vi "Get Assertion Status From Test Case.vi"(11 "Test Case Test Double in":refnum<class "Test Case Test Double.lvclass">) -> (2 "Message":string, 3 "Status":T1)   [LabVIEW 2020, in "LUnit Tests.lvlib" / "Compare Assertion Test.lvclass"]
uses:
  Compare Assertion Test.lvclass
  source/Framework/Result Classes/Assertion Result/Public/TypeDefs/Status.ctl
  Test Dummys/Test Case Test Double/Test Case Test Double.lvclass
  C:/Users/anton/Documents/GitHub/LUnit/source/Framework/Test Case/LUnit Test Case.lvclass
  source/Framework/Test Case/LUnit Test Case.lvclass/LUnit Test Case.ctl
  source/Framework/Result Classes/Test Case Result/Test Case Result.lvclass/Test Case Result.ctl
  source/Framework/Result Classes/Method Result/Method Result.lvclass/Method Result.ctl
  source/Framework/Result Classes/Assertion Result/Assertion Result.lvclass/Assertion Result.ctl
  source/Framework/Test Case/LUnit Test Case.lvclass
  source/Framework/Result Classes/Test Case Result/Test Case Result.lvclass
  source/Framework/Result Classes/Method Result/Method Result.lvclass
  source/Framework/Result Classes/Assertion Result/Assertion Result.lvclass
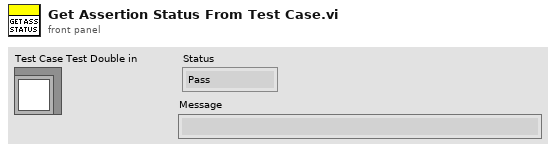
[diagram p1: front panel]
types:
  T1 = typedef "Assertion Result.lvclass/Status.ctl" = enum16{"Pass", "Fail", "Error", "Skipped", "Setup Error", "Broken", "Teardown Error"}
  T2 = map{string, refnum<class "Method Result.lvclass">}
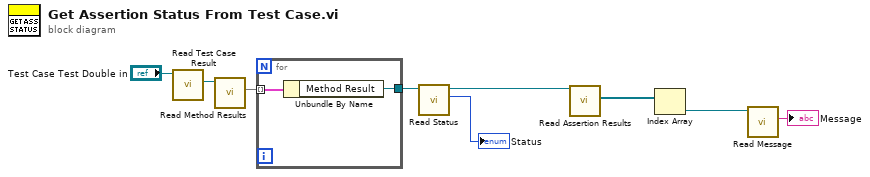
[diagram p0: block diagram]
diagram:
  n1 = call "Read Test Case Result.vi"("LUnit Test Case In"="Test Case Test Double in") -> ("Test Case Result"=w6:refnum<class "Test Case Result.lvclass">)  [unwired: 9 in, 1 out]
  n2 = call "Read Method Results.vi"("Test Case Result In"=w6) -> ("Method Results"=w7:T2)  [unwired: 9 in, 1 out]
  n3 = for {
    tunnel: [w11] -> w8
    tunnel: w7 -> [w10] mode=indexing
    n4 = Unbundle By Name(w10) -> ("Method Result"=w11:refnum<class "Method Result.lvclass">)
  }
  n5 = call "Read Status.vi"("Method Result In"=w8) -> ("Status"=→"Status":T1, "Method Result Out"=w4:refnum<class "Method Result.lvclass">)  [unwired: 8 in, 1 out]
  n6 = call "Read Assertion Results.vi"("Method Result In"=w4) -> ("Assertion Results"=w3:refnum<class "Assertion Result.lvclass">[])  [unwired: 9 in, 1 out]
  n7 = Index Array(array=w3) -> (element=w2:refnum<class "Assertion Result.lvclass">)  [unwired: 1 in]
  n8 = call "Read Message.vi"("Assertion Result In"=w2) -> ("Message"=→"Message":string)  [unwired: 9 in, 1 out]
